vi "oldMain.vi"() -> ()   [LabVIEW 2025]
doc: "Use this template to build a simple state machine design pattern. Each state executes code and determines which state to transition to."
uses:
  <vilib>/Utility/miscctls.llb/LVPoint32TypeDef.ctl
  controls/State.ctl
  controls/Data.ctl
panel:
  out "x-y":T1
  out "y":i32
  out "x":i32
  out "Coords":T2
  in  "page down":bool
  out "pagenum":i32
  in  "page up":bool
  out "timer":timestamp format="%<%H:%M:%S%3u>T"
  out "2D Picture":picture
  out "main tab":T3(tab) caption="Tab Control"
  in  "stop":bool
  in  "Edit entry":bool
  in  "multi entry":bool
  in  "sing entry":bool
  in  "Sp.AI entry":bool
  in  "Countdown entry":bool
  in  "Classic entry":bool
  in  "go back (sel)":bool
  in  "Size (<=25, square)":i32=3 min=3 max=25 step=1
  in  "Layers (<=3)":i32=1 min=1 max=3 step=1
  in  "Toggle barrier":bool
  in  "mapgen sw":bool
  # "map select"
  # "auto gen"
  # "load file"
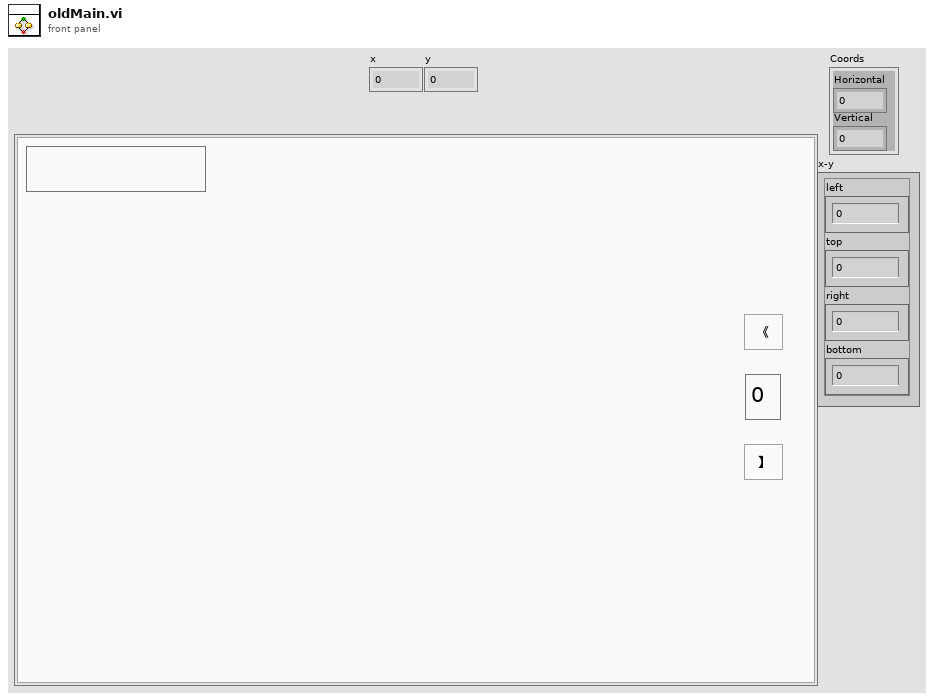
[diagram p1: front panel]
types:
  T1 = cluster{"left":i16, "top":i16, "right":i16, "bottom":i16}
  T2 = typedef "LVPoint32TypeDef.ctl" = cluster{"Horizontal":i32, "Vertical":i32}
  T3 = enum32{"menu", "select page", "sing", "multi", "multi end", "multi setting"}
  T4 = typedef "Data.ctl" = cluster{"barrier":bool, "String <Replace Me>":string, "Numeric <Replace Me>":dbl, "player mode":u16, "mode":u16, "layers":i32, "size":i32}
  T5 = typedef "State.ctl" = enum16{"Initialize", "Menu", "select map", "sing", "multi", "edit", "Exit"}
  T6 = enum8{"Enabled", "Disabled", "Disabled and Grayed Out"}
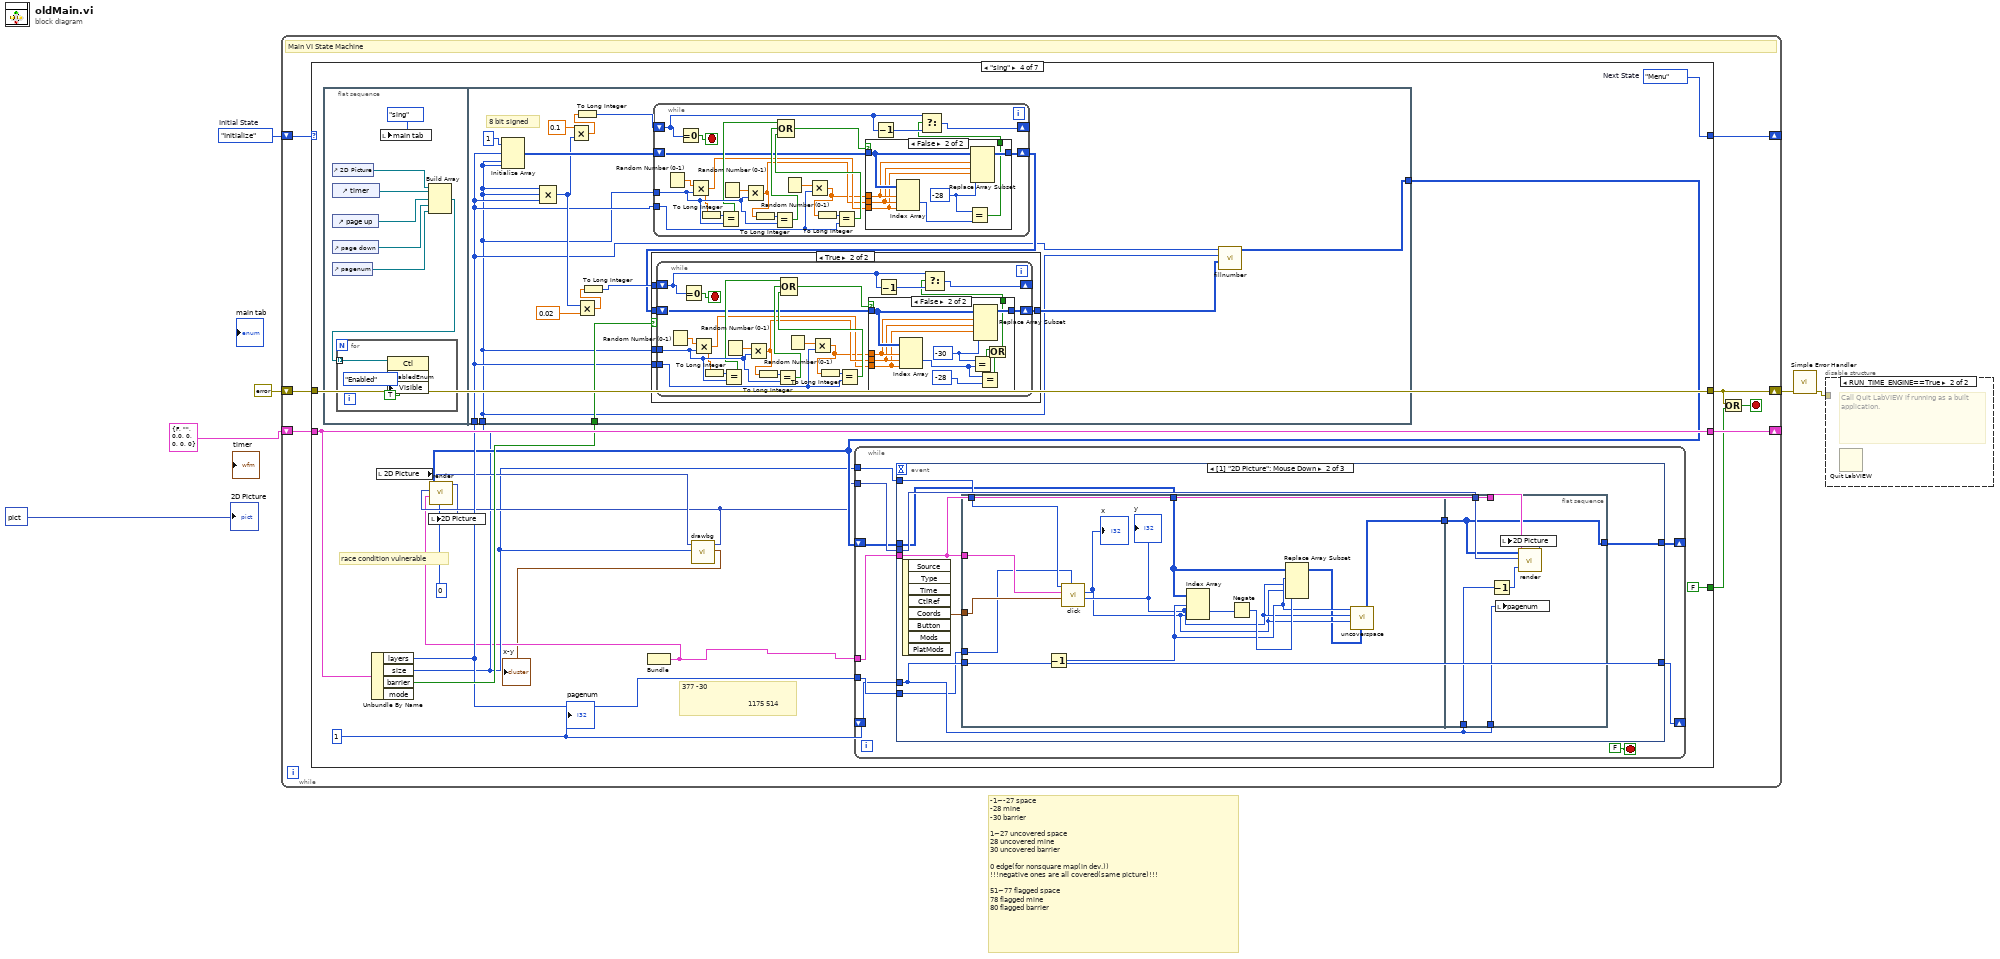
[diagram p0: block diagram]
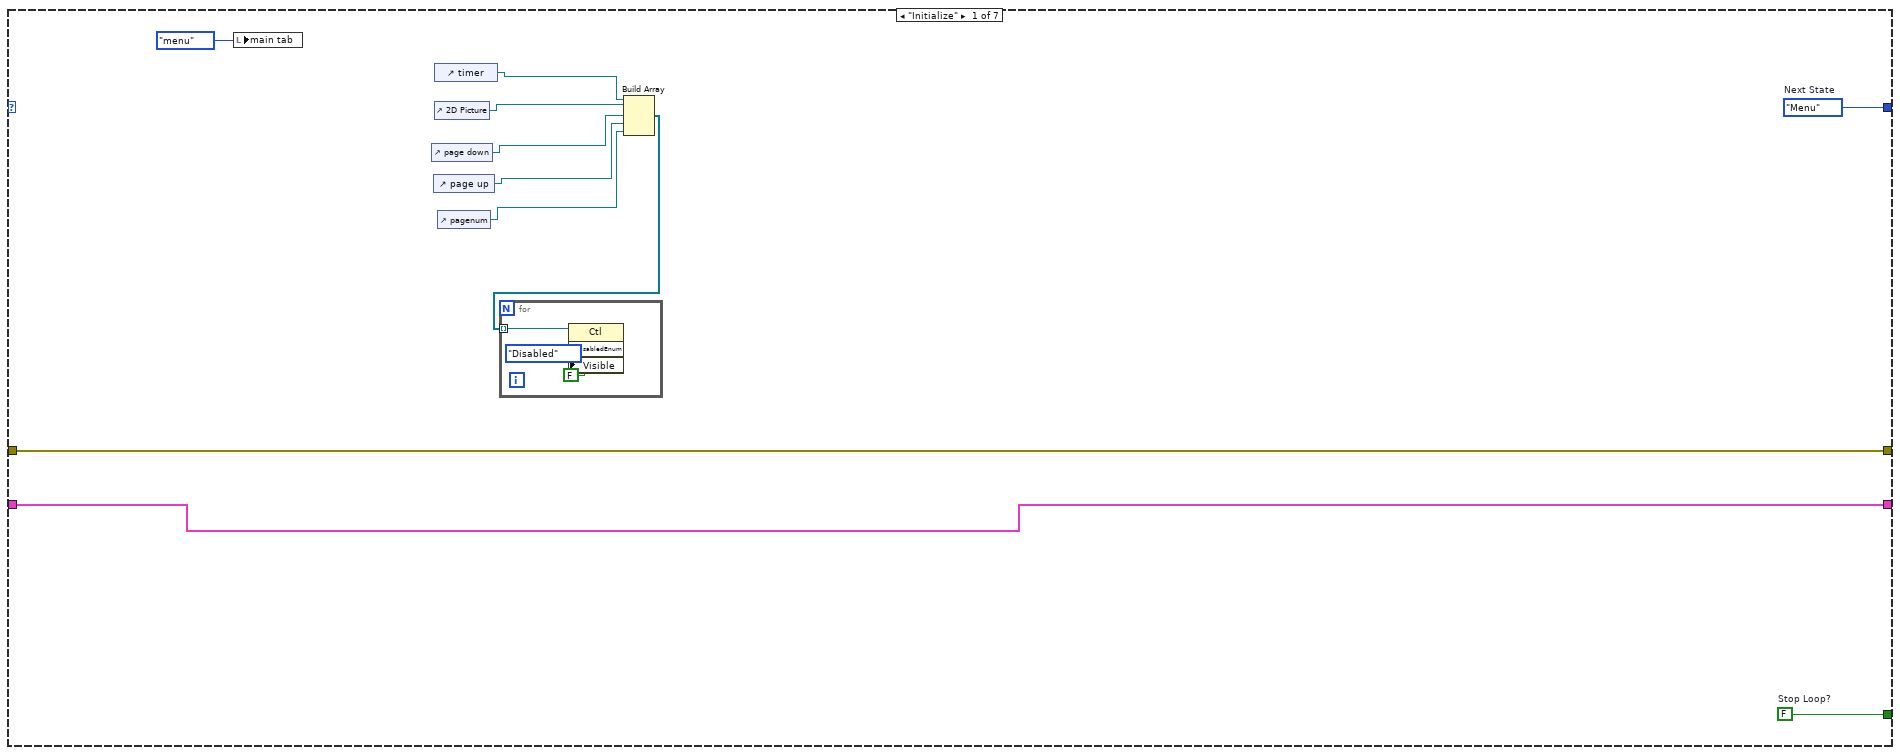
[diagram p3: hidden frame]
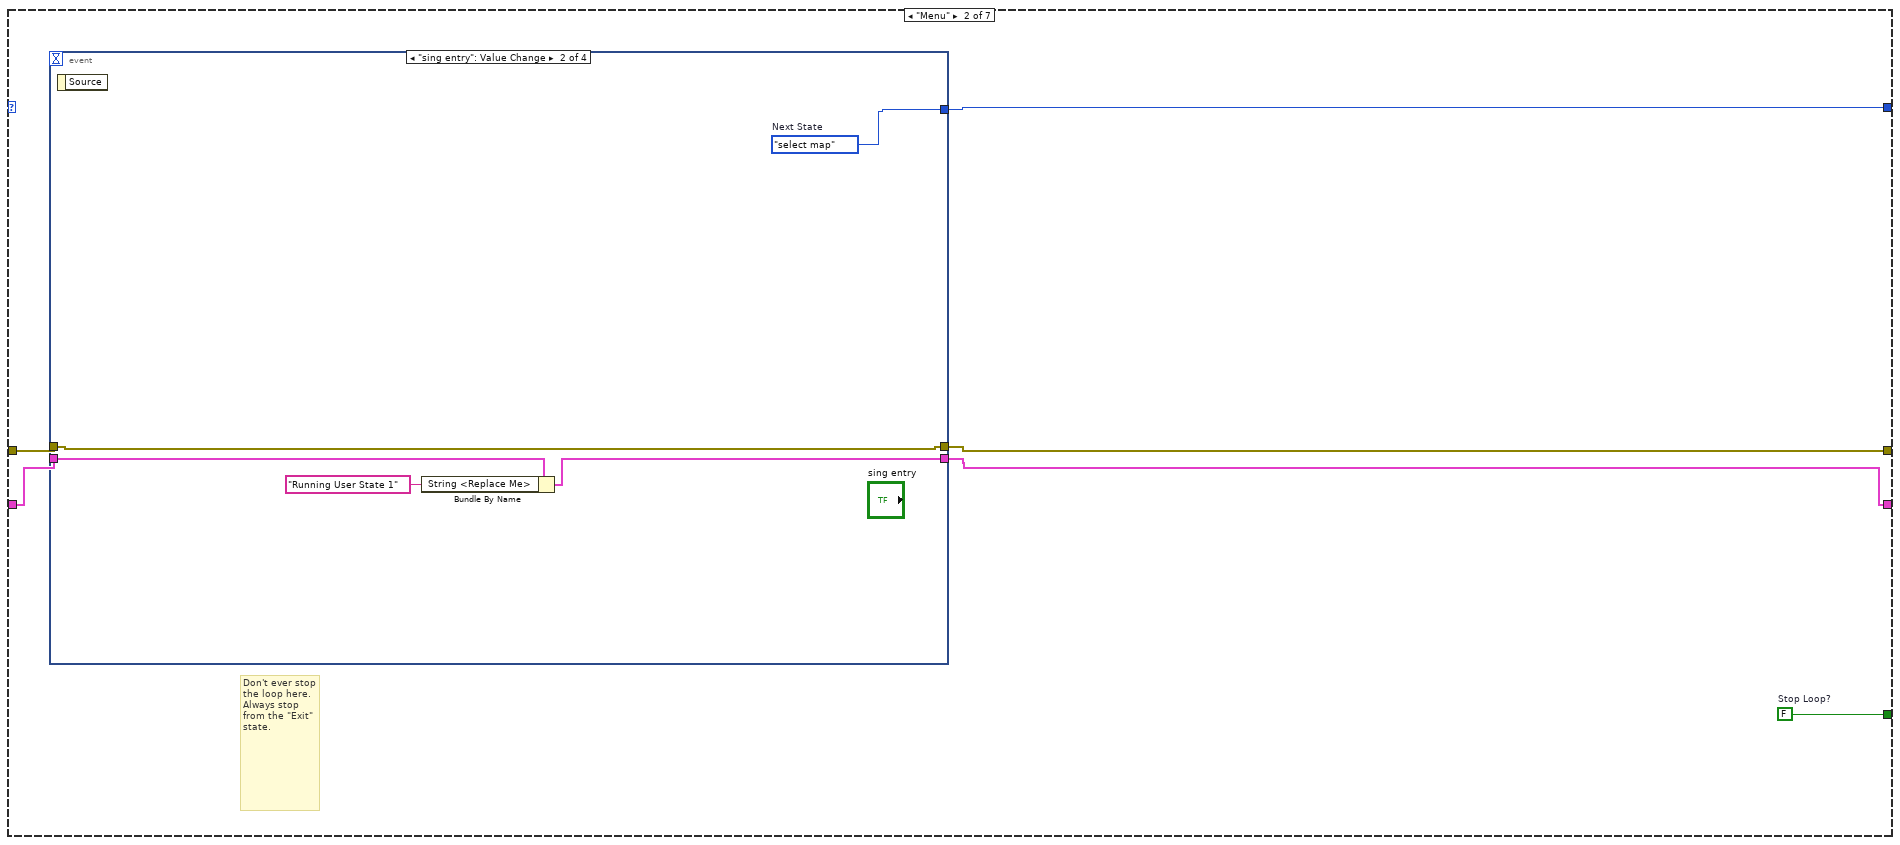
[diagram p4: hidden frame]
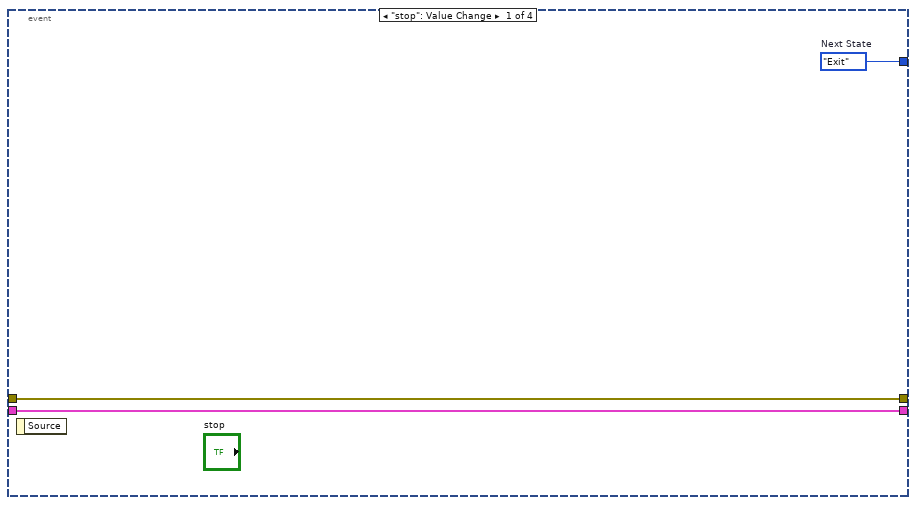
[diagram p5: hidden frame]
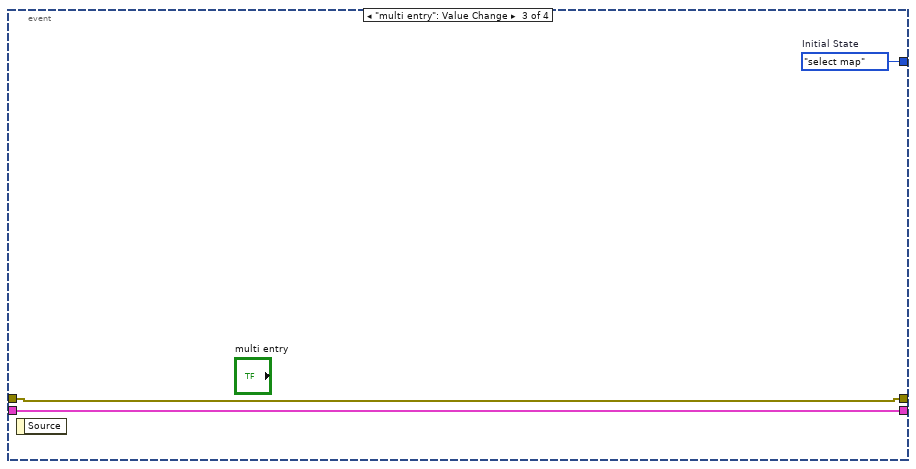
[diagram p6: hidden frame]
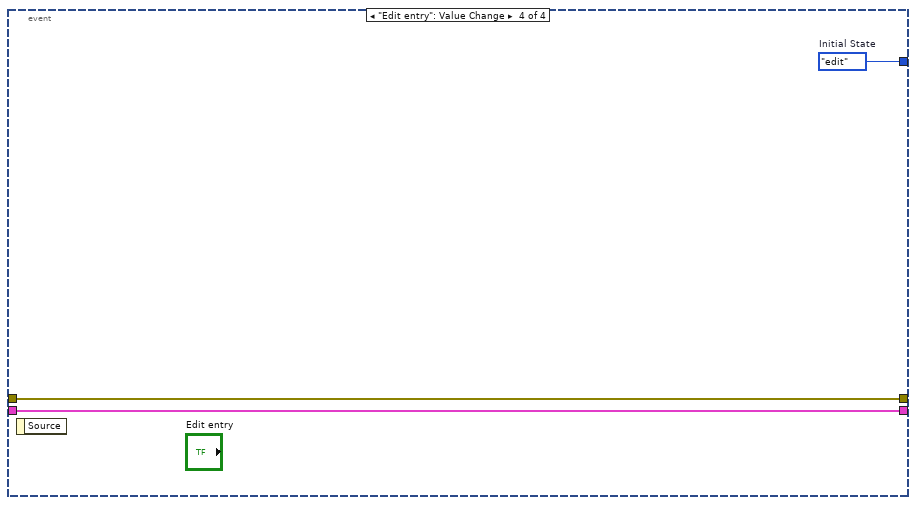
[diagram p7: hidden frame]
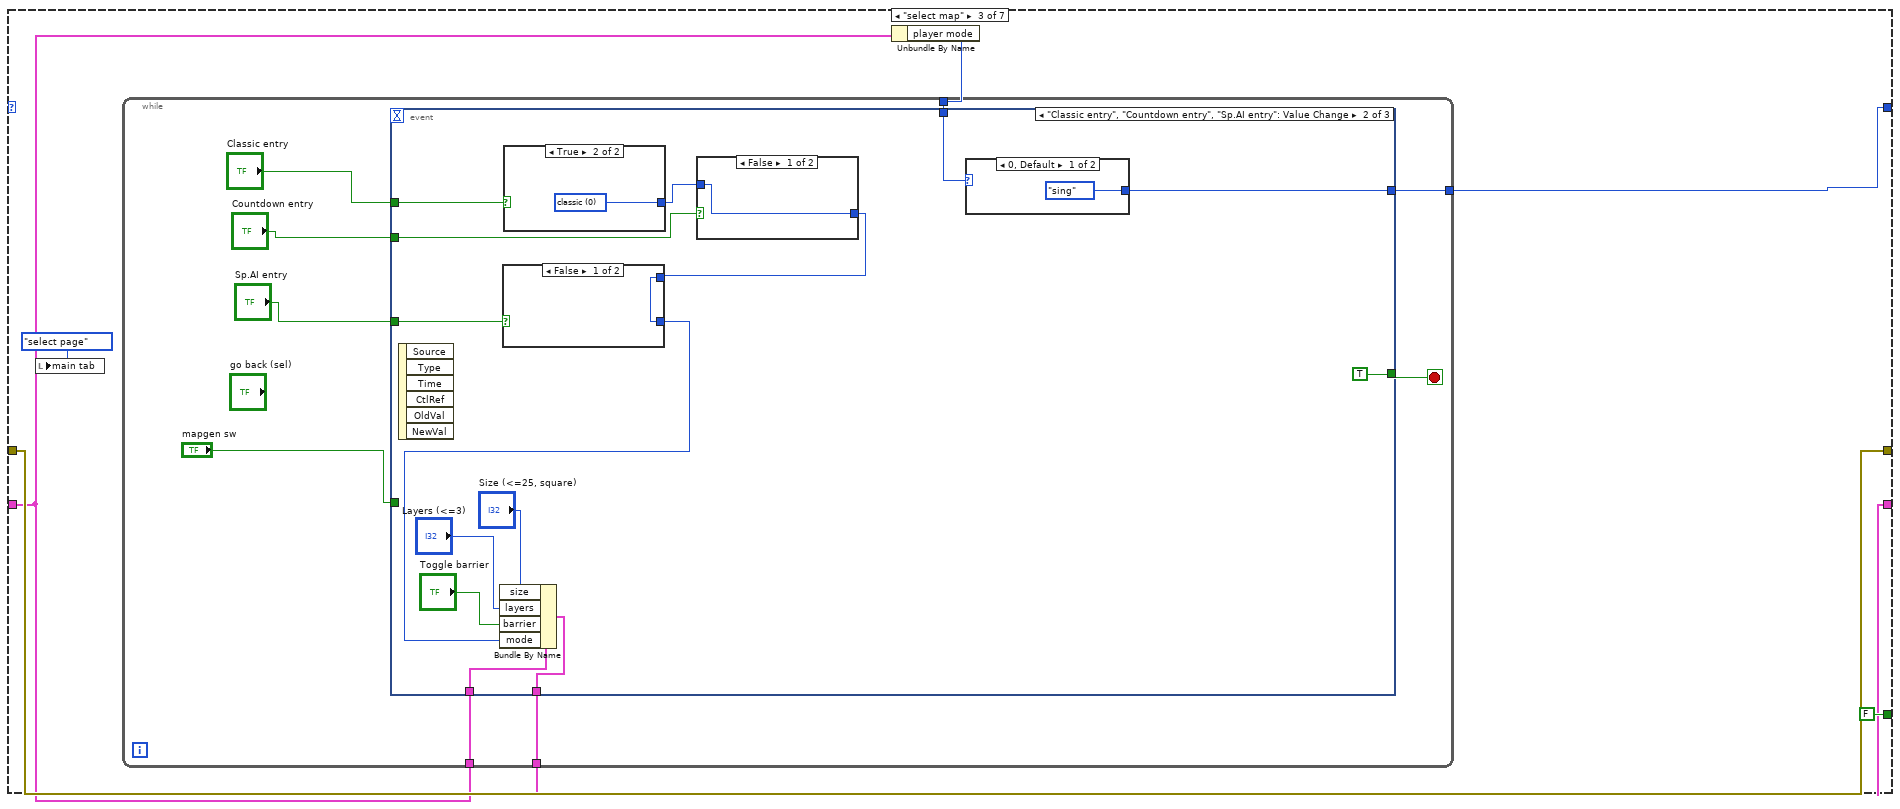
[diagram p8: hidden frame]
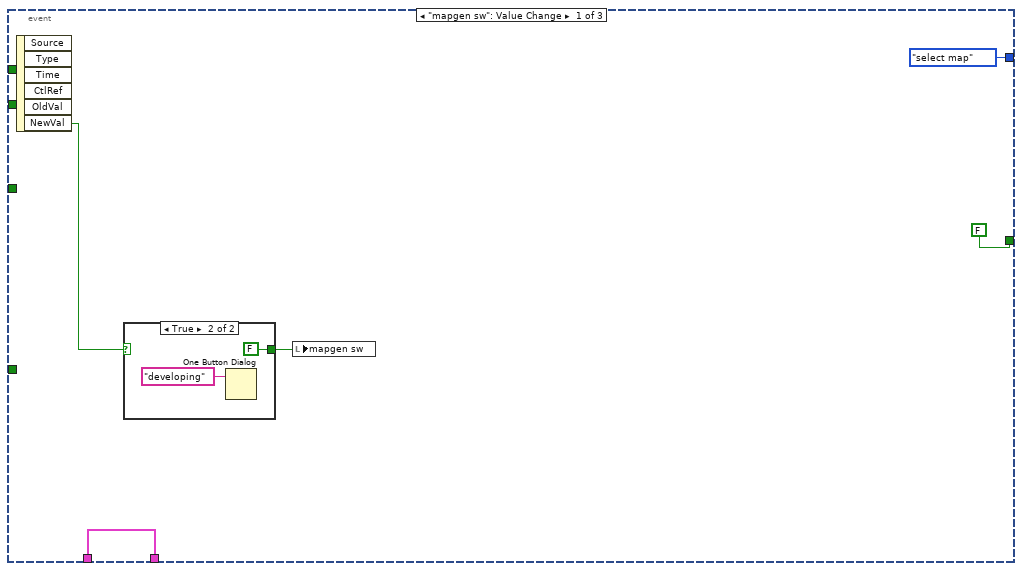
[diagram p9: hidden frame]
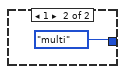
[diagram p11: hidden frame]
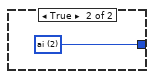
[diagram p12: hidden frame]
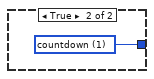
[diagram p13: hidden frame]
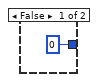
[diagram p14: hidden frame]
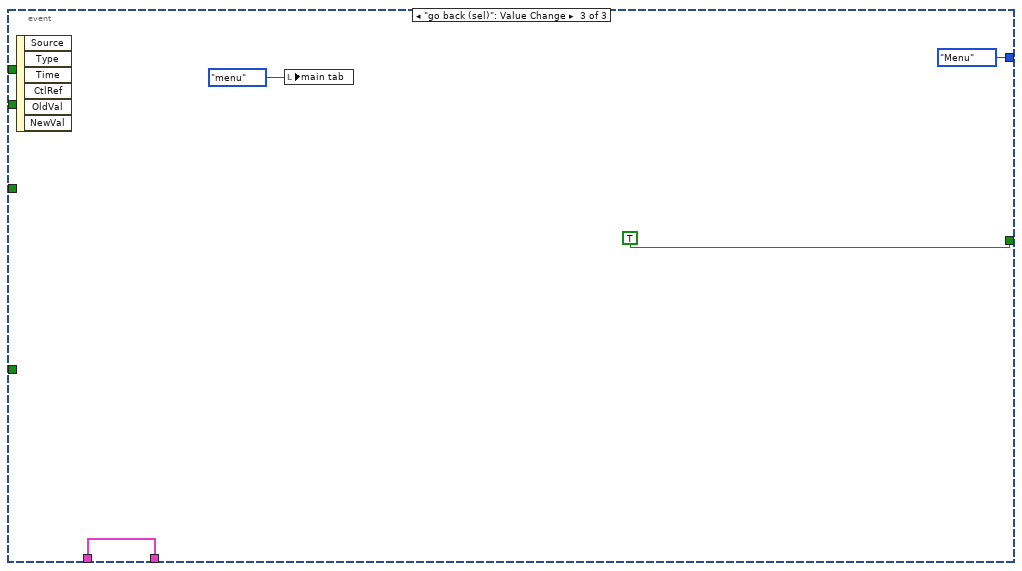
[diagram p15: hidden frame]
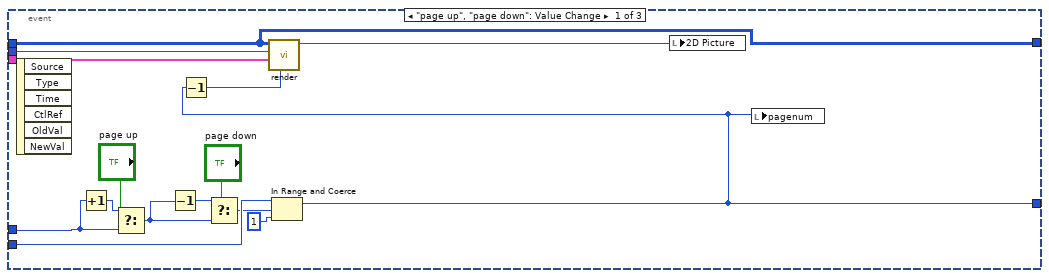
[diagram p16: hidden frame]
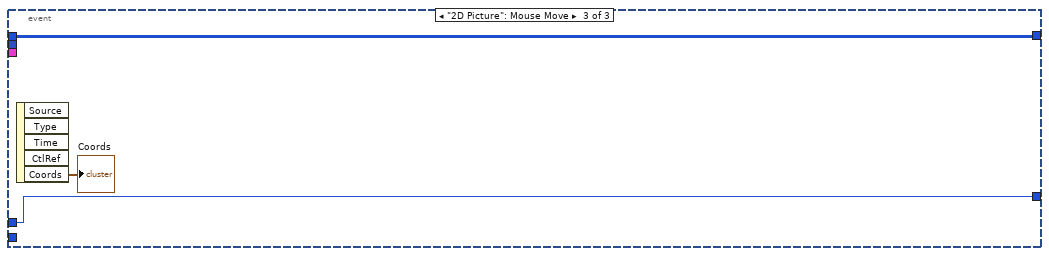
[diagram p17: hidden frame]
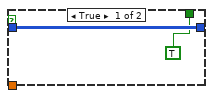
[diagram p19: hidden frame]
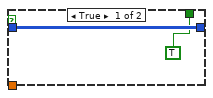
[diagram p20: hidden frame]
diagram:
  w6 = State."Initialize"  # Initial State
  # "-1~-27 space\n-28 mine\n-30 barrier\n\n1~27 uncovered space\n28 uncovered mine\n30 uncovered barrier\n\n0 edge(for nonsquare map(in dev.))\n!!!negative ones are all covered(same picture)!!!\n\n51~77 flagged space\n78 flagged mine\n80 flagged barrier"
  n1 = while {
    shift-right: [w13] -> _
    shift-left: w6 -> [w14]
    shift-right: [w11] -> _
    shift-left: T4 {"barrier"=FALSE, "String <Replace Me>"="", "Numeric <Replace Me>"=0.0, "player mode"=0, "mode"=0, "layers"=0, "size"=0} ("Data") -> [w12]
    shift-right: [w7] -> w4
    shift-left: errorcluster {"status"=FALSE, "code"=0, "source"=""} ("error constant") -> [w10]
    stop <- w8 stop-if-true
    # "Main VI State Machine"
    n2 = case shown="\"sing\"" w14 {
      tunnel: [w25 w34 w49 w113 w272 w274 w284] -> w13
      tunnel: [w24 w33 FALSE ("Stop Loop?") FALSE ("Stop Loop?") FALSE ("Stop Loop?") FALSE ("Stop Loop?") w282] -> w9
      tunnel: w12 -> [w21 w32 w52 w110 w270 w278 w283]
      tunnel: [w21 w31 w53 w110 w270 w278 w283] -> w11
      tunnel: w10 -> [w23 w30 w55 w111 w268 w277 w281]
      tunnel: [w23 w29 w55 w111 w268 w277 w281] -> w7
      frame "Initialize" {
        w24 = FALSE  # Stop Loop?
        w25 = State."Menu"  # Next State
        # "Initialize - Initialize the application."
        n3 = local write "main tab"(T3."menu" ("Tab Control")) -> ()
        n4 = control-ref of="page down"() -> (w17:refnum<vi>)
        n5 = control-ref of="page up"() -> (w16:refnum<vi>)
        n6 = control-ref of="timer"() -> (w19:refnum<vi>)
        n7 = control-ref of="2D Picture"() -> (w18:refnum<vi>)
        n8 = control-ref of="pagenum"() -> (w15:refnum<vi>)
        n9 = Build Array(w19, w18, w17, w16, w15) -> (w20:refnum<vi>[])
        n10 = for {
          tunnel: w20 -> [w26] mode=indexing
          n11 = property on="Property Node" class="Ctl"(reference=w26, "DisabledEnum"=T6."Disabled" ("Disabled"), "Visible"=FALSE) -> ()  [unwired: 1 in, 2 out]
        }
      }
      frame "Menu" {
        w33 = FALSE  # Stop Loop?
        # "Don't ever stop the loop here. Always stop from the \"Exit\" state."
        n12 = event shown="[1] \"sing entry\": Value Change" {
          selector: _ -> [_ _ _ _]
          dyn-events: _ -> [_ _ _ _]
          timeout: _ -> [_ _ _ _]
          tunnel: [w37 w38 w43 w46] -> w34
          tunnel: w32 -> [w36 w42 w45 w48]
          tunnel: [w36 w41 w45 w48] -> w31
          tunnel: w30 -> [w35 w39 w44 w47]
          tunnel: [w35 w39 w44 w47] -> w29
          event "stop": Value Change {
            w37 = State."Exit"  # Next State
            n13 = event-data() -> ()  [unwired: 1 in, 1 out]
          }
          event "sing entry": Value Change {
            w38 = State."select map"  # Next State
            n14 = event-data() -> ()  [unwired: 1 in, 1 out]
            n15 = Bundle By Name(cluster=w42, "String <Replace Me>"="Running User State 1" ("Running User State 1")) -> (w41:T4)
          }
          event "multi entry": Value Change {
            w43 = State."select map"  # Initial State
            n16 = event-data() -> ()  [unwired: 1 in, 1 out]
          }
          event "Edit entry": Value Change {
            w46 = State."edit"  # Initial State
            n17 = event-data() -> ()  [unwired: 1 in, 1 out]
          }
        }
      }
      frame "select map" {
        n18 = local write "main tab"(T3."select page" ("Tab Control")) -> ()
        n19 = Unbundle By Name(w52) -> ("player mode"=w50:u16)
        n20 = while {
          tunnel: w52 -> [w63]
          tunnel: [w62] -> w53
          tunnel: w50 -> [w57]
          tunnel: [w56] -> w49
          stop <- w64 stop-if-true
          n21 = event shown="[1] \"Classic entry\", \"Countdown entry\", \"Sp.AI entry\": Value Change" {
            selector: _ -> [_ _ _]
            dyn-events: _ -> [_ _ _]
            timeout: _ -> [_ _ _]
            tunnel: [FALSE TRUE TRUE] -> w64
            tunnel: w63 -> [w68 w79 w96]
            tunnel: [w68 w80 w96] -> w62
            tunnel: "Classic entry" -> [_ w85 _]
            tunnel: "Countdown entry" -> [_ w84 _]
            tunnel: "Sp.AI entry" -> [_ w81 _]
            tunnel: "mapgen sw" -> [_ _ _]
            tunnel: w57 -> [_ w77 _]
            tunnel: [State."select map" ("(Value Not Used)") w76 State."Menu" ("(Value Not Used)")] -> w56
            event "mapgen sw": Value Change {
              n22 = event-data() -> ("NewVal"=w66:bool)  [unwired: 1 in, 5 out]
              n23 = case shown="True" w66 {
                selector: w66 -> [w70 _]
                tunnel: [w70 FALSE] -> w67
                frame False {
                }
                frame True {
                  n24 = One Button Dialog(message="developing") -> ()  [unwired: 1 in, 1 out]
                }
              }
              n25 = local write "mapgen sw"(w67) -> ()
            }
            event "Classic entry", "Countdown entry", "Sp.AI entry": Value Change {
              n26 = event-data() -> ()  [unwired: 1 in, 6 out]
              n27 = case shown="True" w85 {
                tunnel: [u16 0 w94] -> w83
                frame False {
                }
                frame True {
                  w94 = u16 0 items=["classic", "countdown", "ai"]
                }
              }
              n28 = case shown="False" w84 {
                tunnel: [w91 w92] -> w82
                tunnel: w83 -> [w91 _]
                frame False {
                }
                frame True {
                  w92 = u16 1 items=["classic", "countdown", "ai"]
                }
              }
              n29 = case shown="False" w81 {
                tunnel: [w89 w90] -> w78
                tunnel: w82 -> [w89 _]
                frame False {
                }
                frame True {
                  w90 = u16 2 items=["classic", "countdown", "ai"]
                }
              }
              n30 = Bundle By Name(cluster=w79, "size"="Size (<=25, square)", "layers"="Layers (<=3)", "barrier"="Toggle barrier", "mode"=w78) -> (w80:T4)
              n31 = case shown="0, Default" w77 {
                tunnel: [State."sing" ("(Value Not Used)") State."multi" ("(Value Not Used)")] -> w76
                frame 0, Default {
                }
                frame 1 {
                }
              }
            }
            event "go back (sel)": Value Change {
              n32 = event-data() -> ()  [unwired: 1 in, 6 out]
              n33 = local write "main tab"(T3."menu" ("Tab Control")) -> ()
            }
          }
        }
      }
      frame "sing" {
        w102 = 1
        w113 = State."Menu"  # Next State
        # "race condition vulnerable"
        # "377 -30\n\n                                 1175 514"
        # "User State 1 - Replace this state with functionality for your own application."
        n34 = flat-sequence {
          tunnel: w101 -> [w180]
          tunnel: w108 -> [w181]
          tunnel: w109 -> [w185]
          tunnel: [w182] -> w107
          frame #0 {
            n35 = control-ref of="2D Picture"() -> (w174:refnum<vi>)
            n36 = control-ref of="timer"() -> (w173:refnum<vi>)
            n37 = control-ref of="page up"() -> (w172:refnum<vi>)
            n38 = control-ref of="page down"() -> (w171:refnum<vi>)
            n39 = control-ref of="pagenum"() -> (w170:refnum<vi>)
            n40 = local write "main tab"(T3."sing" ("Tab Control")) -> ()
            n41 = Build Array(w174, w173, w172, w171, w170) -> (w175:refnum<vi>[])
            n42 = for {
              tunnel: w175 -> [w177] mode=indexing
              n43 = property on="Property Node" class="Ctl"(reference=w177, "DisabledEnum"=T6."Enabled" ("Disabled"), "Visible"=TRUE) -> ()  [unwired: 1 in, 2 out]
            }
          }
          frame #1 {
            # "8 bit signed"
            n44 = Initialize Array(i8 1 ("element"), w181, w180, w180) -> (w193:i8[][][])
            n45 = Compound Arithmetic op=MULTIPLY(w180, w180, w181) -> (w184:i32)
            n46 = Multiply(x=0.1 ("y"), y=w184) -> (x*y=w191:dbl)
            n47 = To Long Integer(number=w191) -> (32bit integer=w190:i32)
            n48 = Multiply(x=w184, y=0.02) -> (x*y=w188:dbl)
            n49 = To Long Integer(number=w188) -> (32bit integer=w189:i32)
            n50 = while {
              shift-right: [w257] -> w186
              shift-left: w193 -> [w245]
              tunnel: w181 -> [w246]
              tunnel: w180 -> [w252]
              shift-right: [w239] -> _
              shift-left: w190 -> [w237]
              stop <- w236 stop-if-true
              n51 = Random Number (0-1)() -> (number: 0 to 1=w256:dbl)
              n52 = Equal To 0?(x=w237) -> (x = 0?=w236:bool)
              n53 = Multiply(x=w256, y=w252) -> (x*y=w244:dbl)
              n54 = To Long Integer(number=w244) -> (32bit integer=w254:i32)
              n55 = Equal?(x=w254, y=w252) -> (x = y?=w249:bool)
              n56 = Random Number (0-1)() -> (number: 0 to 1=w255:dbl)
              n57 = Multiply(x=w255, y=w252) -> (x*y=w243:dbl)
              n58 = To Long Integer(number=w243) -> (32bit integer=w253:i32)
              n59 = Equal?(x=w253, y=w252) -> (x = y?=w248:bool)
              n60 = Random Number (0-1)() -> (number: 0 to 1=w250:dbl)
              n61 = Multiply(x=w250, y=w246) -> (x*y=w242:dbl)
              n62 = To Long Integer(number=w242) -> (32bit integer=w251:i32)
              n63 = Equal?(x=w251, y=w246) -> (x = y?=w247:bool)
              n64 = Compound Arithmetic op=OR(w249, w248, w247) -> (w241:bool)
              n65 = case shown="False" w241 {
                tunnel: [w259 w267] -> w257
                tunnel: w245 -> [w259 w266]
                tunnel: w244 -> [_ w260]
                tunnel: w243 -> [_ w261]
                tunnel: w242 -> [_ w262]
                tunnel: [TRUE w263] -> w238
                frame True {
                }
                frame False {
                  w264 = i8 -28 ("element")
                  n66 = Index Array(array=w266, index (dim 0)=w262, index (dim 1)=w261, index (dim 2)=w260) -> (element=w265:i8)
                  n67 = Equal?(x=w264, y=w265) -> (x = y?=w263:bool)
                  n68 = Replace Array Subset(array=w266, new element=w264, index (dim 0)=w262, index (dim 1)=w261, index (dim 2)=w260) -> (w267:i8[][][])
                }
              }
              n69 = Decrement(x=w237) -> (x-1=w240:i32)
              n70 = Select(t=w237, s=w238, f=w240) -> (s? t:f=w239:i32)
            }
            n71 = case shown="True" w185 {
              tunnel: w180 -> [_ w200]
              tunnel: w181 -> [_ w199]
              tunnel: w189 -> [_ w198]
              tunnel: w186 -> [w195 w197]
              tunnel: [w195 w196] -> w183
              frame False {
              }
              frame True {
                n72 = while {
                  shift-right: [w222] -> w196
                  shift-left: w197 -> [w210]
                  tunnel: w199 -> [w211]
                  tunnel: w200 -> [w217]
                  shift-right: [w206] -> _
                  shift-left: w198 -> [w204]
                  stop <- w203 stop-if-true
                  n73 = Random Number (0-1)() -> (number: 0 to 1=w221:dbl)
                  n74 = Equal To 0?(x=w204) -> (x = 0?=w203:bool)
                  n75 = Multiply(x=w221, y=w217) -> (x*y=w202:dbl)
                  n76 = To Long Integer(number=w202) -> (32bit integer=w219:i32)
                  n77 = Equal?(x=w219, y=w217) -> (x = y?=w214:bool)
                  n78 = Random Number (0-1)() -> (number: 0 to 1=w220:dbl)
                  n79 = Multiply(x=w220, y=w217) -> (x*y=w209:dbl)
                  n80 = To Long Integer(number=w209) -> (32bit integer=w218:i32)
                  n81 = Equal?(x=w218, y=w217) -> (x = y?=w213:bool)
                  n82 = Random Number (0-1)() -> (number: 0 to 1=w215:dbl)
                  n83 = Multiply(x=w215, y=w211) -> (x*y=w201:dbl)
                  n84 = To Long Integer(number=w201) -> (32bit integer=w216:i32)
                  n85 = Equal?(x=w216, y=w211) -> (x = y?=w212:bool)
                  n86 = Compound Arithmetic op=OR(w214, w213, w212) -> (w208:bool)
                  n87 = case shown="False" w208 {
                    tunnel: [w224 w235] -> w222
                    tunnel: w210 -> [w224 w234]
                    tunnel: w201 -> [_ w232]
                    tunnel: w209 -> [_ w231]
                    tunnel: w202 -> [_ w230]
                    tunnel: [TRUE w226] -> w205
                    frame True {
                    }
                    frame False {
                      w233 = i8 -30 ("element")
                      n88 = Index Array(array=w234, index (dim 0)=w232, index (dim 1)=w231, index (dim 2)=w230) -> (element=w229:i8)
                      n89 = Equal?(x=w233, y=w229) -> (x = y?=w228:bool)
                      n90 = Replace Array Subset(array=w234, new element=w233, index (dim 0)=w232, index (dim 1)=w231, index (dim 2)=w230) -> (w235:i8[][][])
                      n91 = Equal?(x=w229, y=i8 -28 ("element")) -> (x = y?=w227:bool)
                      n92 = Or(x=w228, y=w227) -> (x .or. y?=w226:bool)
                    }
                  }
                  n93 = Decrement(x=w204) -> (x-1=w207:i32)
                  n94 = Select(t=w204, s=w205, f=w207) -> (s? t:f=w206:i32)
                }
              }
            }
            n95 = call "fillnumber.vi"("map"=w183, "size"=w180, "layers"=w181) -> ("Array out"=w182:i8[][][])  [unwired: 8 in]
          }
        }
        n96 = Unbundle By Name(w110) -> ("layers"=w108:i32, "size"=w101:i32, "barrier"=w109:bool)  [unwired: 1 out]
        n97 = local read "2D Picture"() -> (w106:picture)
        n98 = Bundle() -> (w100:cluster{void, void})  [unwired: 3 in]
        n99 = call "drawbg.vi"("size"=w101, "2D Picture"=w106) -> ("Cluster"=→"x-y":T1, "new picture"=w105:picture)  [unwired: 8 in]
        n100 = call "render.vi"("Numeric"=0, "origin"=w100, "new picture in"=w105, "map"=w107) -> ("new picture out"=w104:picture)  [unwired: 7 in]
        n101 = local write "2D Picture"(w104) -> ()
        n102 = while {
          tunnel: w108 -> [w122]
          tunnel: w100 -> [w121]
          tunnel: w105 -> [w120]
          shift-right: [w118] -> _
          shift-left: w102 -> [w116]
          shift-right: [w115] -> _
          shift-left: w107 -> [w117]
          tunnel: w101 -> [w114]
          stop <- FALSE stop-if-true
          n103 = event shown="[1] \"2D Picture\": Mouse Down" {
            selector: _ -> [_ _ _]
            dyn-events: _ -> [_ _ _]
            timeout: _ -> [_ _ _]
            tunnel: w122 -> [w137 w140 _]
            tunnel: w121 -> [w133 w144 _]
            tunnel: w120 -> [w132 w145 _]
            tunnel: [w124 w141 w169] -> w118
            tunnel: w117 -> [w123 w139 w167]
            tunnel: w116 -> [w125 w141 w169]
            tunnel: [w123 w142 w167] -> w115
            tunnel: w114 -> [_ w143 _]
            event "page up", "page down": Value Change {
              n104 = event-data() -> ()  [unwired: 1 in, 6 out]
              n105 = Increment(x=w125) -> (x+1=w136:i32)
              n106 = Select(t=w136, s="page up", f=w125) -> (s? t:f=w135:i32)
              n107 = Decrement(x=w135) -> (x-1=w134:i32)
              n108 = Select(t=w134, s="page down", f=w135) -> (s? t:f=w130:i32)
              n109 = In Range and Coerce(upper limit=w137, x=w130, lower limit=1) -> (coerced(x)=w124:i32)  [unwired: 1 out]
              n110 = Decrement(x=w124) -> (x-1=w131:i32)
              n111 = call "render.vi"("Numeric"=w131, "origin"=w133, "new picture in"=w132, "map"=w123) -> ("new picture out"=w128:picture)  [unwired: 7 in]
              n112 = local write "2D Picture"(w128) -> ()
              n113 = local write "pagenum"(w124) -> ()
            }
            event "2D Picture": Mouse Down {
              n114 = event-data() -> ("Coords"=w146:T2)  [unwired: 1 in, 7 out]
              n115 = flat-sequence {
                tunnel: w144 -> [w159]
                tunnel: w146 -> [w158]
                tunnel: w143 -> [w157]
                tunnel: w141 -> [w155]
                tunnel: w140 -> [w156]
                tunnel: w139 -> [w154]
                tunnel: [w147] -> w138
                tunnel: w141 -> [w164]
                tunnel: w141 -> [w163]
                tunnel: w144 -> [w162]
                tunnel: w145 -> [w161]
                tunnel: [w160] -> w142
                tunnel: w138 -> [w160]
                frame #0 {
                  n116 = Decrement(x=w155) -> (x-1=w151:i32)
                  n117 = call "click.vi"("page"=w156, "Coords"=w158, "Cluster"=w159, "size"=w157) -> ("y"=w150:i32, "x"=w149:i32)  [unwired: 6 in]
                  "x" <- w149
                  "y" <- w150
                  n118 = Index Array(array=w154, index (dim 0)=w151, index (dim 1)=w150, index (dim 2)=w149) -> (element=w153:i8)
                  n119 = Negate(x=w153) -> (-x=w152:i8)
                  n120 = Replace Array Subset(array=w154, new element=w152, index (dim 0)=w151, index (dim 1)=w150, index (dim 2)=w149) -> (w148:i8[][][])
                  n121 = call "uncoverspace.vi"("input array"=w148, "j"=w149, "i"=w150, "k"=w151) -> ("output array"=w147:i8[][][])  [unwired: 7 in]
                }
                frame #1 {
                  n122 = Decrement(x=w163) -> (x-1=w165:i32)
                  n123 = local write "pagenum"(w164) -> ()
                  n124 = call "render.vi"("Numeric"=w165, "origin"=w162, "new picture in"=w161, "map"=w160) -> ("new picture out"=w166:picture)  [unwired: 7 in]
                  n125 = local write "2D Picture"(w166) -> ()
                }
              }
            }
            event "2D Picture": Mouse Move {
              n126 = event-data() -> ("Coords"=→"Coords":T2)  [unwired: 1 in, 4 out]
            }
          }
        }
        "pagenum" <- w102
      }
      frame "multi" {
        w272 = State."Initialize"  # Next State
        # "User State 2 - Replace this state with functionality for your own application."
        n127 = Unbundle By Name(w270) -> ("String <Replace Me>"=w269:string)
        n128 = One Button Dialog(message=w269) -> ()  [unwired: 1 in, 1 out]
      }
      frame "edit" {
        n129 = One Button Dialog(message="developing") -> (true=w275:bool)  [unwired: 1 in]
        n130 = case shown="False" w275 {
          tunnel: [w279 w280] -> w274
          frame False {
            w279 = State."Menu"  # Initial State
          }
          frame True {
            w280 = State."Menu"  # Initial State
          }
        }
      }
      frame "Exit" {
        w282 = TRUE  # Stop Loop?
        w284 = State."Exit"  # (Value Not Used)
        # "The state value is not used here since this is the last iteration of the state machine loop."
        # "Exit - Exit the application."
      }
    }
    n131 = Or(x=w7, y=w9) -> (x .or. y?=w8:bool)
  }
  n132 = call <vilib>:"Simple Error Handler.vi"("error in (no error)"=w4) -> ("error out"=w3:errorcluster)  [unwired: 4 in, 4 out]
  n133 = disable-structure shown="RUN_TIME_ENGINE==True" {
    disable-tunnel: w3 -> [_ _]
    frame condition #0 (active) {
    }
    frame condition #1 {
      # "Call Quit LabVIEW if running as a built application."
      n134 = Quit LabVIEW() -> ()  [unwired: 1 in]
    }
  }
  "2D Picture" <- picture data[5B] ("2D Picture")
